vi "PWM.vi"() -> ()   [LabVIEW 2016]
uses:
  <vilib>/rvi/Emulation/niFpgaGetClockAttributes.vi
  <vilib>/rvi/Emulation/niFpgaSctlEmulationGetInTimedLoop.vi
  <vilib>/rvi/Emulation/niFpgaEmulationReportErrorSimple.vi
  <vilib>/rvi/eio/common/nirviEmuTemplateMethod_errors.vi
  <vilib>/rvi/Emulation/niFpgaCriticalErrorInLSC.vi
  <vilib>/eio/EIONode/EIONode.xnode
panel:
  out "error out":errorcluster
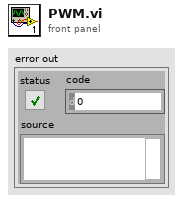
[diagram p1: front panel]
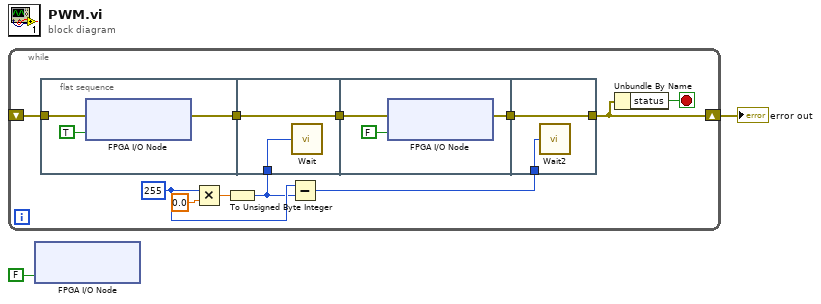
[diagram p0: block diagram]
diagram:
  n1 = while {
    shift-right: [w8] -> w1
    shift-left: _ -> [w9]
    stop <- w10 stop-if-true
    w5 = u8 255 ("x")
    n2 = flat-sequence {
      tunnel: [w15] -> w12
      tunnel: w9 -> [w14]
      tunnel: [w18] -> w13
      tunnel: w12 -> [w18]
      tunnel: w4 -> [w17]
      tunnel: w13 -> [w20]
      tunnel: [w19] -> w11
      tunnel: [w23] -> w8
      tunnel: w11 -> [w23]
      tunnel: w3 -> [w22]
      frame #0 {
        n3 = xnode "FPGA I/O Node"("error in"=w14, "Mod3/DIO1"=TRUE) -> ("error out"=w15:errorcluster)  [unwired: 1 in, 1 out]
      }
      frame #1 {
        n4 = call "Wait"("Count(Ticks)"=w17) -> ()  [unwired: 1 out]
      }
      frame #2 {
        n5 = xnode "FPGA I/O Node"("error in"=w20, "Mod3/DIO1"=FALSE) -> ("error out"=w19:errorcluster)  [unwired: 1 in, 1 out]
      }
      frame #3 {
        n6 = call "Wait2"("Count(Ticks)"=w22) -> ()  [unwired: 1 out]
      }
    }
    n7 = Multiply(x=w5, y=sgl 0.0) -> (x*y=w7:sgl)
    n8 = To Unsigned Byte Integer(number=w7) -> (unsigned 8bit integer=w4:u8)
    n9 = Subtract(x=w5, y=w4) -> (x-y=w3:u8)
    n10 = Unbundle By Name(w8) -> ("status"=w10:bool)
  }
  "error out" <- w1
  n11 = xnode "FPGA I/O Node"("Mod3/DIO2"=FALSE) -> ()  [unwired: 2 in, 2 out]
